vi "delete_license.vi"() -> ()   [LabVIEW 2020]
uses:
  <vilib>/registry/registry.llb/Registry View.ctl
panel:
  in  "addons":T1(array[cluster]) caption="Third-party addons"
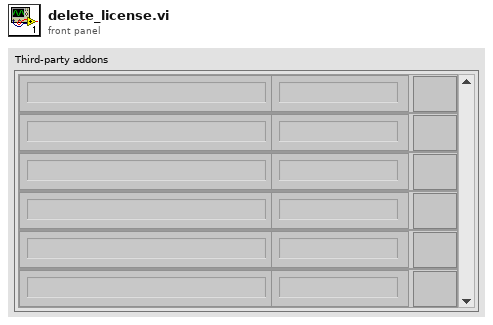
[diagram p1: front panel]
types:
  T1 = cluster{"Addon":string, "Version":string, "Delete":bool}[]
  T2 = typedef "Registry View.ctl" = u16
  T3 = typedef "Registry refnum.ctl" = refnum<k1>
  T4 = cluster{"numSubKeys":i32, "maxSubKeyLen":i32, "maxSubKeyClassLen":i32}
  T5 = cluster{string, "subkey":string, " registry view":T2}
  T6 = cluster{"Addon":string, "Version":string, "Delete":bool}
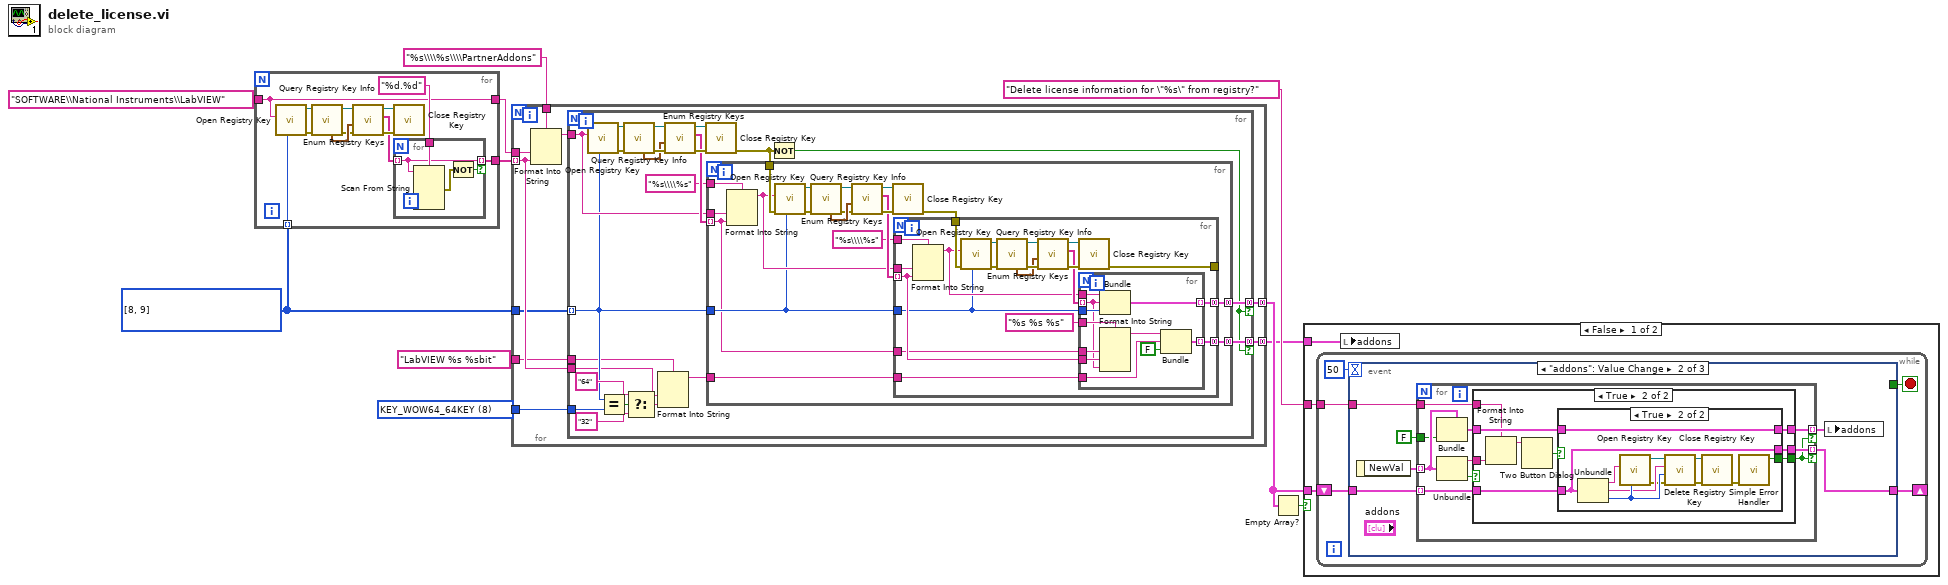
[diagram p0: block diagram]
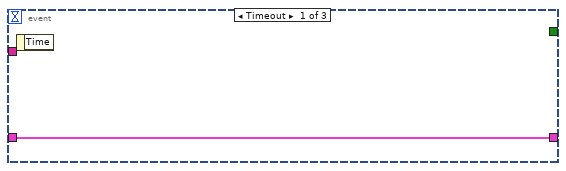
[diagram p2: hidden frame]
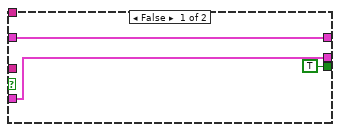
[diagram p3: hidden frame]
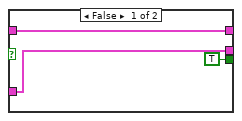
[diagram p4: hidden frame]
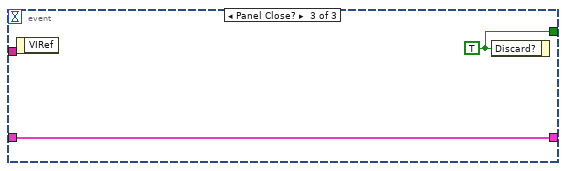
[diagram p5: hidden frame]
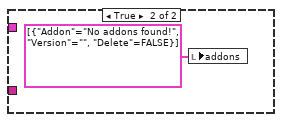
[diagram p6: hidden frame]
diagram:
  w2 = T2 8 items=["Default"=0, "KEY_WOW64_64KEY"=8, "KEY_WOW64_32KEY"=9] ("registry view")
  w5 = T2[] [8, 9] items=["Default"=0, "KEY_WOW64_64KEY"=8, "KEY_WOW64_32KEY"=9] ("registry view")
  n1 = for {
    tunnel: [w14] -> w11
    tunnel: "SOFTWARE\\National Instruments\\LabVIEW" ("subkey") -> [w12]
    tunnel: w5 -> [w13] mode=indexing
    tunnel: [w12] -> w8
    n2 = call <vilib>:"Open Registry Key.vi"("registry view"=w13, "subkey"=w12) -> ("error out"=w22:errorcluster, "refnum out"=w23:T3)  [unwired: 8 in]
    n3 = call <vilib>:"Query Registry Key Info.vi"("error in (no error)"=w22, "refnum"=w23) -> ("error out"=w20:errorcluster, "refnum out"=w19:T3, "subkey info"=w21:T4)  [unwired: 5 in, 2 out]
    n4 = call <vilib>:"Enum Registry Keys.vi"("error in (no error)"=w20, "subkey info"=w21, "refnum"=w19) -> ("error out"=w17:errorcluster, "subkeys"=w16:string[], "refnum out"=w18:T3)  [unwired: 6 in]
    n5 = call <vilib>:"Close Registry Key.vi"("error in (no error)"=w17, "refnum"=w18) -> ()  [unwired: 5 in, 1 out]
    n6 = for {
      tunnel: w16 -> [w26] mode=indexing
      tunnel: "%d.%d" ("format string") -> [w27]
      tunnel: [w26] -> w14 mode=indexing if=w24
      n7 = Scan From String(format string=w27, input string=w26) -> (error out=w25:errorcluster)  [unwired: 6 in, 2 out]
      n8 = Not(x=w25) -> (.not. x?=w24:bool)
    }
  }
  n9 = for {
    tunnel: w11 -> [w32] mode=indexing
    tunnel: w8 -> [w34]
    tunnel: [w36] -> w6 mode=concatenating
    tunnel: "%s\\\\%s\\\\PartnerAddons" ("format string") -> [w35]
    tunnel: w5 -> [w31]
    tunnel: "LabVIEW %s %sbit" ("format string") -> [w30]
    tunnel: w2 -> [w29]
    tunnel: [w28] -> w1 mode=concatenating
    n10 = Format Into String(format string=w35, w34, w32) -> (resulting string=w33:string)  [unwired: 2 in, 1 out]
    n11 = for {
      tunnel: [w39] -> w36 mode=concatenating if=w37
      tunnel: w33 -> [w51]
      tunnel: w31 -> [w45] mode=indexing
      tunnel: w32 -> [w43]
      tunnel: w30 -> [w42]
      tunnel: w29 -> [w41]
      tunnel: [w38] -> w28 mode=concatenating if=w37
      n12 = call <vilib>:"Open Registry Key.vi"("registry view"=w45, "subkey"=w51) -> ("error out"=w53:errorcluster, "refnum out"=w54:T3)  [unwired: 8 in]
      n13 = Equal?(x=w45, y=w41) -> (x = y?=w46:bool)
      n14 = call <vilib>:"Query Registry Key Info.vi"("error in (no error)"=w53, "refnum"=w54) -> ("error out"=w56:errorcluster, "refnum out"=w57:T3, "subkey info"=w55:T4)  [unwired: 5 in, 2 out]
      n15 = Select(t="64", s=w46, f="32") -> (s? t:f=w44:string)
      n16 = Format Into String(format string=w42, w43, w44) -> (resulting string=w40:string)  [unwired: 2 in, 1 out]
      n17 = call <vilib>:"Enum Registry Keys.vi"("error in (no error)"=w56, "subkey info"=w55, "refnum"=w57) -> ("error out"=w59:errorcluster, "subkeys"=w52:string[], "refnum out"=w58:T3)  [unwired: 6 in]
      n18 = call <vilib>:"Close Registry Key.vi"("error in (no error)"=w59, "refnum"=w58) -> ("error out"=w49:errorcluster)  [unwired: 5 in]
      n19 = for {
        tunnel: w52 -> [w63] mode=indexing
        tunnel: w45 -> [w66]
        tunnel: w51 -> [w77]
        tunnel: "%s\\\\%s" ("format string") -> [w78]
        tunnel: w49 -> [w69]
        tunnel: w40 -> [w62]
        tunnel: [w61] -> w39 mode=concatenating
        tunnel: [w60] -> w38 mode=concatenating
        n20 = Format Into String(format string=w78, w77, w63) -> (resulting string=w67:string)  [unwired: 2 in, 1 out]
        n21 = call <vilib>:"Open Registry Key.vi"("registry view"=w66, "error in (no error)"=w69, "subkey"=w67) -> ("error out"=w76:errorcluster, "refnum out"=w75:T3)  [unwired: 7 in]
        n22 = call <vilib>:"Query Registry Key Info.vi"("error in (no error)"=w76, "refnum"=w75) -> ("error out"=w73:errorcluster, "refnum out"=w72:T3, "subkey info"=w74:T4)  [unwired: 5 in, 2 out]
        n23 = call <vilib>:"Enum Registry Keys.vi"("error in (no error)"=w73, "subkey info"=w74, "refnum"=w72) -> ("error out"=w70:errorcluster, "subkeys"=w68:string[], "refnum out"=w71:T3)  [unwired: 6 in]
        n24 = call <vilib>:"Close Registry Key.vi"("error in (no error)"=w70, "refnum"=w71) -> ("error out"=w65:errorcluster)  [unwired: 5 in]
        n25 = for {
          tunnel: w68 -> [w86] mode=indexing
          tunnel: w67 -> [w91]
          tunnel: w66 -> [w80]
          tunnel: w65 -> [w90]
          tunnel: "%s\\\\%s" ("format string") -> [w89]
          tunnel: w63 -> [w85]
          tunnel: w62 -> [w84]
          tunnel: [w82] -> w61 mode=concatenating
          tunnel: [w81] -> w60 mode=concatenating
          tunnel: [w79] -> _
          n26 = Format Into String(format string=w89, w91, w86) -> (resulting string=w83:string)  [unwired: 2 in, 1 out]
          n27 = call <vilib>:"Open Registry Key.vi"("registry view"=w80, "error in (no error)"=w90, "subkey"=w83) -> ("error out"=w92:errorcluster, "refnum out"=w93:T3)  [unwired: 7 in]
          n28 = call <vilib>:"Query Registry Key Info.vi"("error in (no error)"=w92, "refnum"=w93) -> ("error out"=w95:errorcluster, "refnum out"=w96:T3, "subkey info"=w94:T4)  [unwired: 5 in, 2 out]
          n29 = call <vilib>:"Enum Registry Keys.vi"("error in (no error)"=w95, "subkey info"=w94, "refnum"=w96) -> ("error out"=w98:errorcluster, "subkeys"=w88:string[], "refnum out"=w97:T3)  [unwired: 6 in]
          n30 = call <vilib>:"Close Registry Key.vi"("error in (no error)"=w98, "refnum"=w97) -> ("error out"=w79:errorcluster)  [unwired: 5 in]
          n31 = for {
            tunnel: w88 -> [w100] mode=indexing
            tunnel: "%s %s %s" ("format string") -> [w109]
            tunnel: w86 -> [w108]
            tunnel: w85 -> [w107]
            tunnel: w84 -> [w104]
            tunnel: w83 -> [w99]
            tunnel: [w102] -> w82 mode=indexing
            tunnel: [w103] -> w81 mode=indexing
            tunnel: w80 -> [w101]
            n32 = Bundle(w99, "subkey"=w100, "registry view"=w101) -> (w102:T5)  [unwired: 1 in]
            n33 = Format Into String(format string=w109, w107, w108, w100) -> (resulting string=w105:string)  [unwired: 2 in, 1 out]
            n34 = Bundle(w105, w104, FALSE) -> (w103:cluster{string, string, bool})  [unwired: 1 in]
          }
        }
      }
      n35 = Not(x=w49) -> (.not. x?=w37:bool)
    }
  }
  n36 = Empty Array?(array=w6) -> (empty?=w7:bool)
  n37 = case shown="False" w7 {
    tunnel: w6 -> [w112 _]
    tunnel: "Delete license information for \"%s\" from registry?" -> [w111 _]
    tunnel: w1 -> [w110 _]
    frame False {
      n38 = while {
        tunnel: w111 -> [w115]
        shift-right: [w114] -> _
        shift-left: w112 -> [w116]
        stop <- w113 stop-if-true
        n39 = event shown="[1] \"addons\": Value Change" {
          selector: _ -> [_ _ _]
          dyn-events: _ -> [_ _ _]
          timeout: 50 -> [_ _ _]
          tunnel: w116 -> [w118 w123 w162]
          tunnel: w115 -> [_ w122 _]
          tunnel: [w118 w120 w162] -> w114
          tunnel: [_ _ w161] -> w113
          event Timeout {
            n40 = event-data() -> ()  [unwired: 1 in, 1 out]
          }
          event "addons": Value Change {
            n41 = event-data() -> ("NewVal"=w124:T1)  [unwired: 1 in]
            n42 = for {
              tunnel: w124 -> [w128] mode=indexing
              tunnel: w123 -> [w132] mode=indexing
              tunnel: w122 -> [w125]
              tunnel: [w131] -> w121 mode=indexing if=w129
              tunnel: [w130] -> w120 mode=indexing if=w129
              tunnel: FALSE -> [w127]
              n43 = Bundle(cluster=w128, "Delete"=w127) -> (w126:T6)  [unwired: 2 in]
              n44 = Unbundle(w128) -> ("Addon"=w133:string, "Delete"=w134:bool)  [unwired: 1 out]
              n45 = case shown="True" w134 {
                tunnel: w133 -> [_ w146]
                tunnel: w132 -> [w137 w143]
                tunnel: [w137 w142] -> w130
                tunnel: [w135 w141] -> w131
                tunnel: [TRUE w140] -> w129
                tunnel: w126 -> [w135 w139]
                tunnel: w125 -> [_ w138]
                frame False {
                }
                frame True {
                  n46 = Format Into String(format string=w138, w146) -> (resulting string=w145:string)  [unwired: 2 in, 1 out]
                  n47 = Two Button Dialog(message=w145) -> (T button?=w144:bool)  [unwired: 2 in]
                  n48 = case shown="True" w144 {
                    tunnel: w143 -> [w148 w155]
                    tunnel: w139 -> [w149 w154]
                    tunnel: [w148 w155] -> w142
                    tunnel: [w149 w154] -> w141
                    tunnel: [TRUE w153] -> w140
                    frame False {
                    }
                    frame True {
                      n49 = Unbundle(w155) -> (w152:string, "subkey"=w151:string, "registry view"=w159:T2)
                      n50 = call <vilib>:"Open Registry Key.vi"("registry view"=w159, "subkey"=w152) -> ("error out"=w150:errorcluster, "refnum out"=w160:T3)  [unwired: 8 in]
                      n51 = call <vilib>:"Delete Registry Key.vi"("error in (no error)"=w150, "registry view"=w159, "subkey"=w151, "refnum"=w160) -> ("error out"=w157:errorcluster, "refnum out"=w158:T3)  [unwired: 6 in]
                      n52 = call <vilib>:"Close Registry Key.vi"("error in (no error)"=w157, "refnum"=w158) -> ("error out"=w156:errorcluster)  [unwired: 5 in]
                      n53 = call <vilib>:"Simple Error Handler.vi"("error in (no error)"=w156) -> ("error?"=w153:bool)  [unwired: 4 in, 4 out]
                    }
                  }
                }
              }
            }
            n54 = local write "addons"(w121) -> ()
          }
          event Panel Close? {
            w161 = TRUE ("Discard?")
            n55 = event-data() -> ()  [unwired: 1 in, 1 out]
            n56 = event-data("Discard?"=w161) -> ()  [unwired: 1 in, 1 out]
          }
        }
      }
      n57 = local write "addons"(w110) -> ()
    }
    frame True {
      n58 = local write "addons"(T1 [{"Addon"="No addons found!", "Version"="", "Delete"=FALSE}] ("addons")) -> ()
    }
  }
